vi "Get_All_Files_In_Folder.vi"(4 "length":i32=1, 6 "offset (for subset of folder)":i32, 8 "error in (no error)":errorcluster, 11 "File or Folder Path":path=path "C:/") -> (0 "error out":errorcluster, 1 "pattern":string="*.dat", 3 "array of files":path[](array[path]))   [LabVIEW 2016]
uses:
  <userlib>/LevyLab/LV to ITX/LVtoITX.lvclass
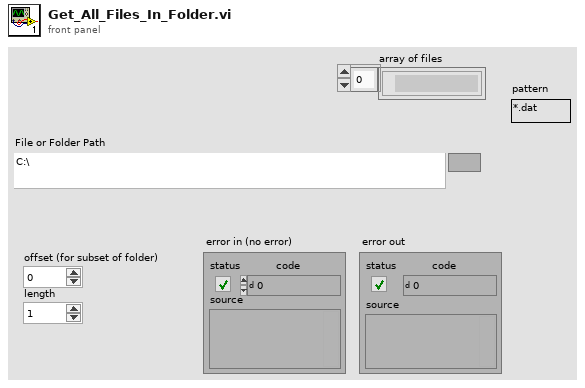
[diagram p1: front panel]
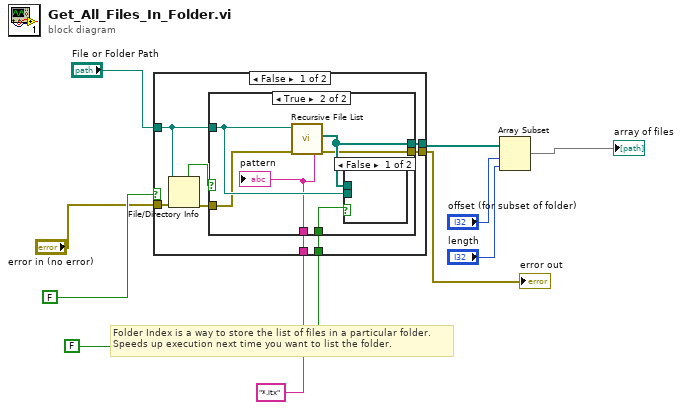
[diagram p0: block diagram]
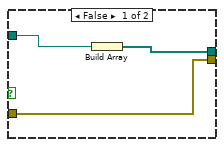
[diagram p2: hidden frame]
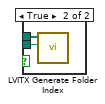
[diagram p3: hidden frame]
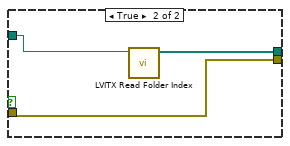
[diagram p4: hidden frame]
diagram:
  # "Folder Index is a way to store the list of files in a particular folder.\nSpeeds up execution next time you want to list the folder."
  n1 = case shown="False" FALSE ("Use Folder Index File?") {
    tunnel: [w16 w31] -> w5
    tunnel: "File or Folder Path" -> [w18 w32]
    tunnel: FALSE ("Generate Folder Index File?") -> [w15 _]
    tunnel: "*.itx" ("pattern") -> [w14 _]
    tunnel: "error in (no error)" -> [w13 w30]
    tunnel: [w11 w30] -> w1
    frame False {
      n2 = File/Directory Info(path=w18, error in=w13) -> (directory=w17:bool, error out=w12:errorcluster)  [unwired: 5 out]
      n3 = case shown="True" w17 {
        tunnel: [w21 w25] -> w16
        tunnel: w18 -> [w20 w27]
        tunnel: w15 -> [_ w26]
        tunnel: w14 -> [_ w24]
        tunnel: w12 -> [w19 w23]
        tunnel: [w19 w22] -> w11
        frame False {
          n4 = Build Array(w20) -> (w21:path[])
        }
        frame True {
          n5 = call <vilib>:"Recursive File List.vi"("pattern"=w24, "error in (no error)"=w23, "Folder Path"=w27) -> ("error out"=w22:errorcluster, "All Files in Dir"=w25:path[])  [unwired: 4 in, 3 out]
          n6 = case shown="False" w26 {
            tunnel: w25 -> [_ w29]
            tunnel: w27 -> [_ w28]
            frame False {
            }
            frame True {
              n7 = call <userlib>:"LVITX Generate Folder Index.vi"("File or Folder Path"=w28, "All Files in Dir"=w29) -> ()  [unwired: 10 in]
            }
          }
          "pattern" <- w24
        }
      }
    }
    frame True {
      n8 = call <userlib>:"LVITX Read Folder Index.vi"("File or Folder Path"=w32) -> ("Array"=w31:path[])  [unwired: 10 in]
    }
  }
  "error out" <- w1
  n9 = Array Subset(array=w5, index="offset (for subset of folder)", length="length") -> (→"array of files":path[])
